vi "targeted_sensory_dynamics_v2.vi"() -> ()   [LabVIEW 2014]
uses:
  <vilib>/vision/Measure.llb/Straight Edge Options.ctl
  <vilib>/vision/Measure.llb/Straight Edge Process.ctl
  <vilib>/Platform/TimedLoop/XDataNode/timing_clust.ctl
  <vilib>/Platform/TimedLoop/XDataNode/nitl_modes.ctl
  <vilib>/Platform/TimedLoop/XDataNode/wakeup.ctl
  <vilib>/vision/Measure.llb/Edge Options.ctl
  <vilib>/vision/Measure.llb/Edge Polarity.ctl
  <vilib>/DAQmx/create/channels.llb/DAQmx Create Channel (DO-Digital Output).vi
  <vilib>/DAQmx/write.llb/DAQmx Write (Digital Bool 1Line 1Point).vi
  <vilib>/gmath/statdist.llb/Uniform (Discrete) Random.vi
  <vilib>/DAQmx/create/channels.llb/DAQmx Create Channel (AO-Voltage-Basic).vi
  <vilib>/Platform/TimedLoop/TimeConversion.llb/rt-rel-time-to-milliseconds.vi
  <vilib>/DAQmx/write.llb/DAQmx Write (Analog DBL 1Chan 1Samp).vi
  <vilib>/DAQmx/create/channels.llb/DAQmx Create Channel (DI-Digital Input).vi
  <vilib>/DAQmx/read.llb/DAQmx Read (Digital Bool 1Line 1Point).vi
  <vilib>/platform/TimedLoop/XDataNode/XDataNode.xnode
  <vilib>/vision/driver/NI_Vision_Acquisition_Software.lvlib
  <vilib>/Platform/TimedLoop/XDataNode/XDNodeRunTimeDep.lvlib
  <vilib>/vision/NI_Vision_Development_Module.lvlib
  <vilib>/gmath/NI_Gmath.lvlib
panel:
  out "Trial Light":dbl
  out "Light Trial?":bool=TRUE
  out "Slide 7":dbl(slide) scale=0.0..1.0
  out "Slide 6":dbl(slide) scale=0.0..1.0
  out "W, 90":i32
  out "M, 90":i32
  in  "Light Intensity (V)":dbl=3.9 format="%#_13g"
  in  "Wind Intensity (V)":dbl=3.7 format="%#_13g"
  out "Wind Trial?":bool=TRUE
  out "Initial Orientation":dbl
  out "Slide 5":dbl(slide) scale=0.0..1.0
  out "Slide 4":dbl(slide) scale=0.0..1.0
  out "Slide 3":dbl(slide) scale=0.0..1.0
  out "Slide 2":dbl(slide) scale=0.0..1.0
  out "V, 90":i32
  out "W, 0":i32
  out "M, 0":i32
  out "V, 0":i32
  in  "Reversed Tether?":bool=TRUE
  in  "R options":T1={"Number of Lines"=1, "Type"=enum."Best Edge Projection", "Min. Score"=10.0, "Max. Score"=1000.0, "Orientation"=-135.0, "Angle Range"=45.0, "Angle Tolerance"=1.0, "Step Size"=3, "Min. SNR (db)"=0.0, "Min. Points (%)"=25.0, "Hough Iterations"=3} {"Min. Points (%)" min=0.0 max=100.0; "Min. SNR (db)" min=0.0; "Max. Score" min=0.0 max=1024.0; "Min. Score" min=0.0 max=1024.0 step=1.0}
  in  "L options":T1={"Number of Lines"=1, "Type"=enum."Best Edge Projection", "Min. Score"=10.0, "Max. Score"=1000.0, "Orientation"=135.0, "Angle Range"=45.0, "Angle Tolerance"=1.0, "Step Size"=3, "Min. SNR (db)"=0.0, "Min. Points (%)"=25.0, "Hough Iterations"=3} {"Min. Points (%)" min=0.0 max=100.0; "Min. SNR (db)" min=0.0; "Max. Score" min=0.0 max=1024.0; "Min. Score" min=0.0 max=1024.0 step=1.0}
  out "X (steps/sample)":dbl(graph)
  out "Slide":dbl(slide) scale=0.0..1.0
  out "Motor Error":bool
  in  "Max steps/sample":dbl=6.0
  in  "Step Rate (Hz)":dbl=500.0
  out "Heading (deg)":dbl(graph)
  out "H":dbl format="%.4f"
  out "X (steps/sample)":dbl
  in  "Geneotype":string="w+ Canton-S"
  in  "Starvation Time (hrs)":string="1"
  in  "Age (DSE)":string="4"
  out "Trial End":bool
  in  "Trial Duration (s)":dbl=25.0
  out "Trial":i32 format="%#.3f"
  in  "Number of Trials":i32=30
  in  "Experiment name":string="E1"
  in  "Fly ID":string
  in  "L-R WBA Offset (deg)":dbl format="%#_13g"
  in  "deltaWBA Scale Factor (k, unitless)":dbl=0.04 format="%.4f"
  out "L-R WBA":dbl
  out "deltaWBA":dbl format="%.4f"
  out "Scaled deltaWBA (deg)":dbl(graph)
  out "R WBA":dbl
  out "L WBA":dbl
  out "Image":T3(plugin-control)
  in  "Image Threshold":cluster{"Lower value":sgl, "Upper value":sgl}={"Lower value"=110.0, "Upper value"=255.0} {"Upper value" format="%.2f"; "Lower value" format="%.2f"}
  in  "Data Rate (Hz)":dbl=50.0
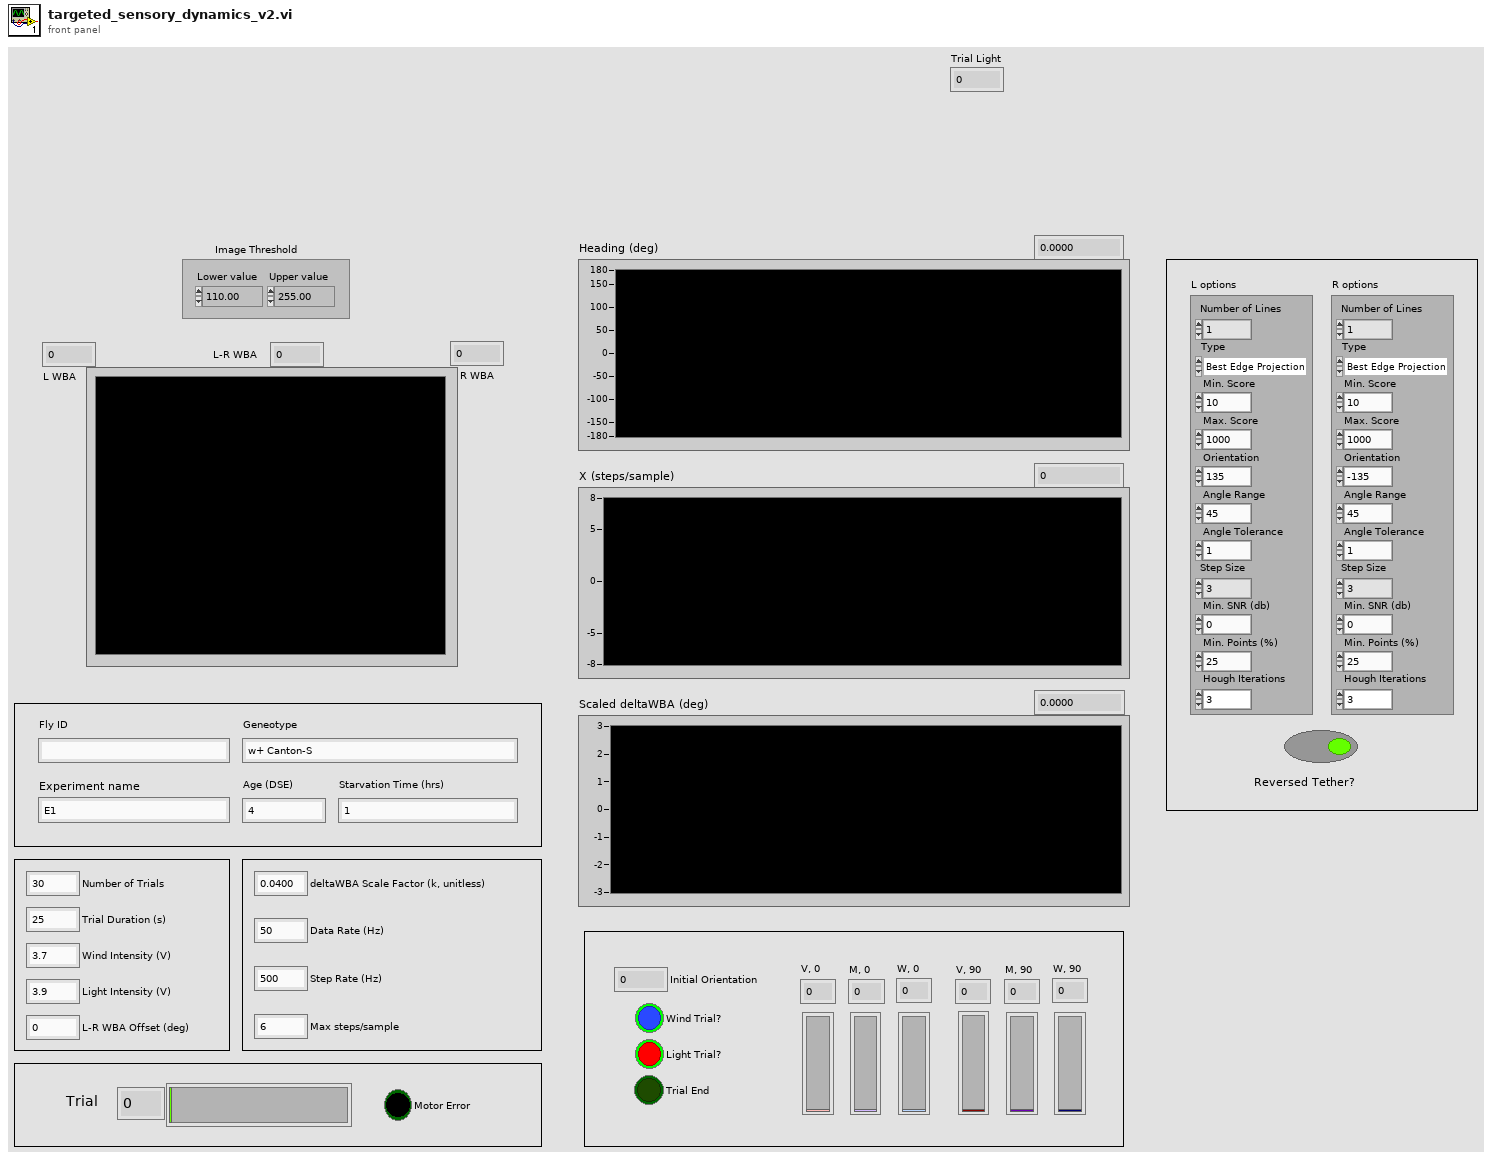
[diagram p1: front panel]
types:
  T1 = typedef "Straight Edge Options.ctl" = cluster{"Number of Lines":i32, "Type":T2, "Min. Score":dbl, "Max. Score":dbl, "Orientation":dbl, "Angle Range":dbl, "Angle Tolerance":dbl, "Step Size":u32, "Min. SNR (db)":dbl, "Min. Points (%)":dbl, "Hough Iterations":i32}
  T2 = typedef "Straight Edge Process.ctl" = enum32{"First Edge Rake", "Best Edge Rake", "Hough Edge Rake", "First Edge Projection", "Best Edge Projection"}
  T3 = typedef "IMAQ Image.ctl" = refnum<image>
  T4 = enum16{"open", "replace", "create", "open or create", "replace or create", "replace or create with confirmation"}
  T5 = typedef "IMAQdx.ctl" = refnum<k21>
  T6 = typedef "IMAQ Rectangle" = cluster{"Left":i32, "Top":i32, "Right":i32, "Bottom":i32, "Rotation":dbl}
  T7 = typedef "ROI Descriptor" = cluster{"Global Rectangle":i32[], "Contours":cluster{"ID":enum32{"External", "Internal"}, "Type":u32, "Coordinates":i32[]}[]}
  T8 = typedef "XDNodeRunTimeDep.lvlib/timing_clust.ctl" = cluster{"Expected End [f-1]":u64, "Actual End [f-1]":u64, "Finished Late? [f-1]":bool, "Expected End [i-1]":u64, "Actual End [i-1]":u64, "Finished Late? [i-1]":bool, "Expected Start [i]":u64, "Actual Start [i]":u64, "Expected Start [f]":u64, "Actual Start [f]":u64, "Source Name":string, "Structure Name":string, "Period":i64, "Deadline":i64, "Offset":i64, "Start":i64, "Priority":i32, "Timeout":i32, "Mode":T9, "Wakeup Reason":T10, "Error":errorcluster, "Source Type":string, "Secondary Source Type":string, "Global End Time":u64, "Global Start Time":u64, "Frame Duration":u64, "Iteration Duration":u64, "Assigned CPU":i32, "I/O Scan Engine Mode":u32}
  T9 = typedef "XDNodeRunTimeDep.lvlib/nitl_modes.ctl" = enum32{"No Change", "Process missed periods, maintain original phase", "Discard missed periods, maintain original phase", "Process missed periods, ignore original phase", "Discard missed periods, ignore original phase"}
  T10 = typedef "XDNodeRunTimeDep.lvlib/wakeup.ctl" = enum32{"Normal", "Aborted", "Asynchronous wakeup", "Timing source error", "Timed loop error", "Timeout"}
  T11 = cluster{"y":i32, "y":i32, "y":i32, "y":i32, "y":i32, "y":i32}
  T12 = typedef "Edge Options.ctl" = cluster{"Edge Polarity":T13, "Kernel Size":u32, "Width":u32, "Minimum Edge Strength":sgl, "Interpolation Type":enum32{"Zero Order", "Bilinear", "Quadratic", "Cubic", "Bilinear Fixed"}, "Data Processing Method":enum32{"Average", "Median"}}
  T13 = typedef "Edge Polarity.ctl" = u32
  T14 = cluster{"Search Direction":u32, "Edge Options":T12, "Show Search Area":bool, "Show Search Lines":bool, "Show Edges Found":bool, "Show Result":bool, "Search Area Color":u32, "Search Lines Color":u32, "Edge Locations Color":u32, "Result Color":u32, "Overlay Group Name":string}
  T15 = cluster{"Point1 (Pixels)":cluster{"X":sgl, "Y":sgl}, "Point2 (Pixels)":cluster{"X":sgl, "Y":sgl}, "Point1 (Real-World)":cluster{"X":sgl, "Y":sgl}, "Point2 (Real-World)":cluster{"X":sgl, "Y":sgl}, "Angle (Pixel)":dbl, "Angle (Real-World)":dbl, "Score":dbl, "Straightness":dbl, "Average SNR (db)":dbl, "Calibration Valid":bool}[]
  T16 = cluster{"Straight Edges[0]":cluster{"Point1 (Pixels)":cluster{"X":sgl, "Y":sgl}, "Point2 (Pixels)":cluster{"X":sgl, "Y":sgl}, "Point1 (Real-World)":cluster{"X":sgl, "Y":sgl}, "Point2 (Real-World)":cluster{"X":sgl, "Y":sgl}, "Angle (Pixel)":dbl, "Angle (Real-World)":dbl, "Score":dbl, "Straightness":dbl, "Average SNR (db)":dbl, "Calibration Valid":bool}, "Straight Edges[1]":cluster{"Point1 (Pixels)":cluster{"X":sgl, "Y":sgl}, "Point2 (Pixels)":cluster{"X":sgl, "Y":sgl}, "Point1 (Real-World)":cluster{"X":sgl, "Y":sgl}, "Point2 (Real-World)":cluster{"X":sgl, "Y":sgl}, "Angle (Pixel)":dbl, "Angle (Real-World)":dbl, "Score":dbl, "Straightness":dbl, "Average SNR (db)":dbl, "Calibration Valid":bool}, "Straight Edges[2]":cluster{"Point1 (Pixels)":cluster{"X":sgl, "Y":sgl}, "Point2 (Pixels)":cluster{"X":sgl, "Y":sgl}, "Point1 (Real-World)":cluster{"X":sgl, "Y":sgl}, "Point2 (Real-World)":cluster{"X":sgl, "Y":sgl}, "Angle (Pixel)":dbl, "Angle (Real-World)":dbl, "Score":dbl, "Straightness":dbl, "Average SNR (db)":dbl, "Calibration Valid":bool}, "Straight Edges[3]":cluster{"Point1 (Pixels)":cluster{"X":sgl, "Y":sgl}, "Point2 (Pixels)":cluster{"X":sgl, "Y":sgl}, "Point1 (Real-World)":cluster{"X":sgl, "Y":sgl}, "Point2 (Real-World)":cluster{"X":sgl, "Y":sgl}, "Angle (Pixel)":dbl, "Angle (Real-World)":dbl, "Score":dbl, "Straightness":dbl, "Average SNR (db)":dbl, "Calibration Valid":bool}, "Straight Edges[4]":cluster{"Point1 (Pixels)":cluster{"X":sgl, "Y":sgl}, "Point2 (Pixels)":cluster{"X":sgl, "Y":sgl}, "Point1 (Real-World)":cluster{"X":sgl, "Y":sgl}, "Point2 (Real-World)":cluster{"X":sgl, "Y":sgl}, "Angle (Pixel)":dbl, "Angle (Real-World)":dbl, "Score":dbl, "Straightness":dbl, "Average SNR (db)":dbl, "Calibration Valid":bool}, "Straight Edges[5]":cluster{"Point1 (Pixels)":cluster{"X":sgl, "Y":sgl}, "Point2 (Pixels)":cluster{"X":sgl, "Y":sgl}, "Point1 (Real-World)":cluster{"X":sgl, "Y":sgl}, "Point2 (Real-World)":cluster{"X":sgl, "Y":sgl}, "Angle (Pixel)":dbl, "Angle (Real-World)":dbl, "Score":dbl, "Straightness":dbl, "Average SNR (db)":dbl, "Calibration Valid":bool}, "Straight Edges[6]":cluster{"Point1 (Pixels)":cluster{"X":sgl, "Y":sgl}, "Point2 (Pixels)":cluster{"X":sgl, "Y":sgl}, "Point1 (Real-World)":cluster{"X":sgl, "Y":sgl}, "Point2 (Real-World)":cluster{"X":sgl, "Y":sgl}, "Angle (Pixel)":dbl, "Angle (Real-World)":dbl, "Score":dbl, "Straightness":dbl, "Average SNR (db)":dbl, "Calibration Valid":bool}, "Straight Edges[7]":cluster{"Point1 (Pixels)":cluster{"X":sgl, "Y":sgl}, "Point2 (Pixels)":cluster{"X":sgl, "Y":sgl}, "Point1 (Real-World)":cluster{"X":sgl, "Y":sgl}, "Point2 (Real-World)":cluster{"X":sgl, "Y":sgl}, "Angle (Pixel)":dbl, "Angle (Real-World)":dbl, "Score":dbl, "Straightness":dbl, "Average SNR (db)":dbl, "Calibration Valid":bool}, "Straight Edges[8]":cluster{"Point1 (Pixels)":cluster{"X":sgl, "Y":sgl}, "Point2 (Pixels)":cluster{"X":sgl, "Y":sgl}, "Point1 (Real-World)":cluster{"X":sgl, "Y":sgl}, "Point2 (Real-World)":cluster{"X":sgl, "Y":sgl}, "Angle (Pixel)":dbl, "Angle (Real-World)":dbl, "Score":dbl, "Straightness":dbl, "Average SNR (db)":dbl, "Calibration Valid":bool}}
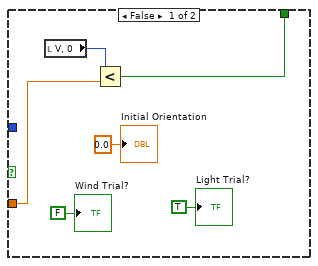
[diagram p2: hidden frame]
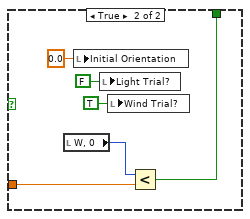
[diagram p3: hidden frame]
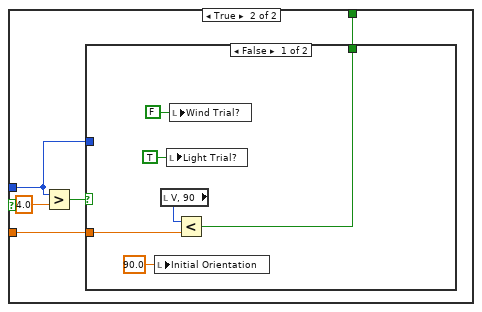
[diagram p4: hidden frame]
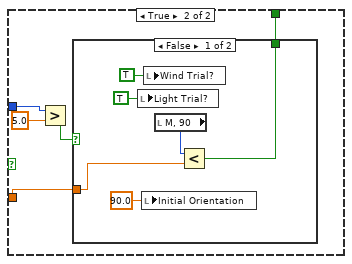
[diagram p5: hidden frame]
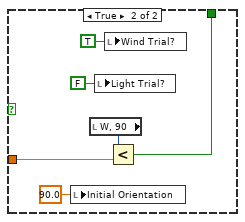
[diagram p6: hidden frame]
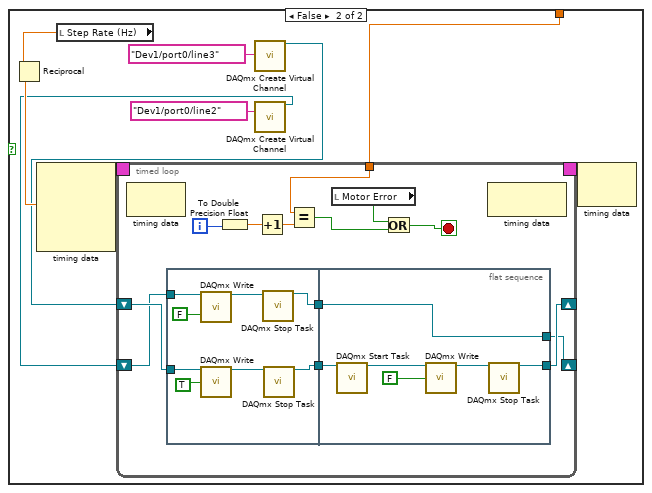
[diagram p8: hidden frame]
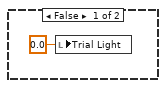
[diagram p9: hidden frame]
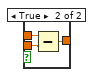
[diagram p11: hidden frame]
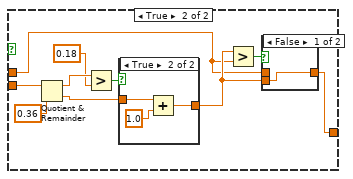
[diagram p15: hidden frame]
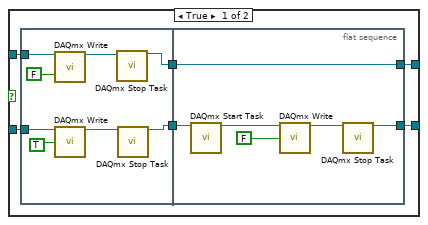
[diagram p19: hidden frame]
diagram:
  w83 = "."
  w85 = "."
  n1 = local read "Wind Intensity (V)"() -> (w21:dbl)
  n2 = local read "deltaWBA Scale Factor (k, unitless)"() -> (w63:dbl)
  n3 = local read "Data Rate (Hz)"() -> (w64:dbl)
  n4 = local read "Trial Duration (s)"() -> (w69:dbl)
  n5 = local read "Number of Trials"() -> (w71:i32)
  n6 = local read "Light Intensity (V)"() -> (w19:dbl)
  n7 = local read "Max steps/sample"() -> (w61:dbl)
  n8 = local read "Step Rate (Hz)"() -> (w62:dbl)
  n9 = local read "Reversed Tether?"() -> (w43:bool)
  n10 = Boolean To (0,1)(Boolean=w43) -> (0, 1=w44:i16)
  n11 = To Double Precision Float(number=w44) -> (double precision float=w42:dbl)
  n12 = Number To Fractional String(number=w19, precision (6)=i16 3) -> (F-format string=w17:string)  [unwired: 2 in]
  n13 = Number To Fractional String(number=w71, precision (6)=i16 0) -> (F-format string=w55:string)  [unwired: 2 in]
  n14 = Number To Fractional String(number=w69, precision (6)=i16 0) -> (F-format string=w54:string)  [unwired: 2 in]
  n15 = Number To Fractional String(number=w21, precision (6)=i16 3) -> (F-format string=w18:string)  [unwired: 2 in]
  n16 = Number To Fractional String(number=w64, precision (6)=i16 0) -> (F-format string=w16:string)  [unwired: 2 in]
  n17 = Number To Fractional String(number=w62, precision (6)=i16 0) -> (F-format string=w15:string)  [unwired: 2 in]
  n18 = Number To Fractional String(number=w61, precision (6)=i16 0) -> (F-format string=w14:string)  [unwired: 2 in]
  n19 = Number To Fractional String(number=w63, precision (6)=i16 3) -> (F-format string=w13:string)  [unwired: 2 in]
  n20 = Number To Fractional String(number=w42, precision (6)=i16 0) -> (F-format string=w12:string)  [unwired: 2 in]
  n21 = Get Date/Time In Seconds() -> (seconds since 1Jan1904=w91:timestamp)
  n22 = Get Date/Time In Seconds() -> (seconds since 1Jan1904=w87:timestamp)
  n23 = Get Date/Time In Seconds() -> (seconds since 1Jan1904=w89:timestamp)
  n24 = call <vilib>:"Space Constant.vi"() -> ("String"=w93:string)
  n25 = Format Date/Time String(time format string (%c)="%d", seconds (now)=w91) -> (date/time string=w82:string)  [unwired: 1 in]
  n26 = Format Date/Time String(time format string (%c)="%m", seconds (now)=w89) -> (date/time string=w84:string)  [unwired: 1 in]
  n27 = Format Date/Time String(time format string (%c)="%Y", seconds (now)=w87) -> (date/time string=w86:string)  [unwired: 1 in]
  n28 = Concatenate Strings(w86, w85, w84, w83, w82) -> (w60:string)
  n29 = Concatenate Strings(w86, w85, w84, w83, w82, w93, "fly_", "Fly ID", "\\") -> (w97:string)
  n30 = String To Path(string=w97) -> (path=w96:path)
  n31 = Build Path(base path=path "E:/TAC DATA ARCHIVE/NewRig/labview/ClosedLoop+OpenWindLightOdor", name or relative path=w96) -> (appended path=w101:path)
  n32 = call <vilib>:"IMAQdx Open Camera.vi"("Session In"=refnum<k21> "cam8" ("Camera Name")) -> ("Session Out"=w123:T5)  [unwired: 2 in, 8 out]
  n33 = call <vilib>:"Check if File or Folder Exists.vi"("path"=w101) -> ("file or folder exists?"=w99:bool, "dup path"=w100:path)  [unwired: 8 in, 1 out]
  n34 = call <vilib>:"IMAQdx Configure Grab.vi"("Session In"=w123) -> ("Session Out"=w121:T5)  [unwired: 1 in, 9 out]
  n35 = case shown="False" w99 {
    tunnel: w100 -> [w125 w126]
    tunnel: [w124 w126] -> w105
    frame False {
      n36 = Create Folder(path (use dialog)=w125) -> (created path=w124:path)  [unwired: 2 in, 2 out]
    }
    frame True {
    }
  }
  n37 = call "IMAQ Create"("Image Name"="ROIR") -> ("New Image"=w120:T3)  [unwired: 3 in, 2 out]
  n38 = Concatenate Strings("Experiment name", "\\") -> (w73:string)
  n39 = call <vilib>:"IMAQdx Grab.vi"("Image In"=w120, "Session In"=w121) -> ("Image Out"=w119:T3, "Session Out"=w110:T5)  [unwired: 2 in, 6 out]
  n40 = String To Path(string=w73) -> (path=w102:path)
  n41 = call "IMAQ Select Rectangle"("Prompt"="Select RIGHT ROI for wing angle detection", "Image In"=w119) -> ("Rectangle"=w111:T6)  [unwired: 6 in, 3 out]
  n42 = Build Path(base path=w105, name or relative path=w102) -> (appended path=w106:path)
  n43 = call "IMAQ Convert Rectangle to ROI"("Rectangle"=w111) -> ("ROI Descriptor"=w109:T7)  [unwired: 8 in, 1 out]
  n44 = call <vilib>:"Check if File or Folder Exists.vi"("path"=w106) -> ("file or folder exists?"=w103:bool, "dup path"=w104:path)  [unwired: 8 in, 1 out]
  n45 = call "IMAQ Create"("Image Name"="ROIL") -> ("New Image"=w115:T3)  [unwired: 3 in, 2 out]
  n46 = case shown="False" w103 {
    tunnel: w104 -> [w128 w129]
    tunnel: [w127 w129] -> w6
    frame False {
      n47 = Create Folder(path (use dialog)=w128) -> (created path=w127:path)  [unwired: 2 in, 2 out]
    }
    frame True {
    }
  }
  n48 = call <vilib>:"IMAQdx Grab.vi"("Image In"=w115, "Session In"=w110) -> ("Image Out"=w114:T3, "Session Out"=w108:T5)  [unwired: 2 in, 6 out]
  n49 = String To Path(string="experiment_information") -> (path=w81:path)
  n50 = call "IMAQ Select Rectangle"("Prompt"="Select LEFT ROI for wing angle detection", "Image In"=w114) -> ("Rectangle"=w116:T6)  [unwired: 6 in, 3 out]
  n51 = Build Path(base path=w6, name or relative path=w81) -> (appended path=w78:path)
  n52 = String To Path(string="initial_orientations") -> (path=w31:path)
  n53 = String To Path(string="wind_boolean") -> (path=w52:path)
  n54 = String To Path(string="light_boolean") -> (path=w10:path)
  n55 = call "IMAQ Convert Rectangle to ROI"("Rectangle"=w116) -> ("ROI Descriptor"=w107:T7)  [unwired: 8 in, 1 out]
  n56 = Build Path(base path=w6, name or relative path=w31) -> (appended path=w28:path)
  n57 = Build Path(base path=w6, name or relative path=w52) -> (appended path=w49:path)
  n58 = Build Path(base path=w6, name or relative path=w10) -> (appended path=w8:path)
  n59 = Open/Create/Replace File(file path (use dialog)=w78, operation (0:open)=T4."create", access (0:read/write)=enum16{"read/write", "read-only", "write-only"}."write-only") -> (refnum out=w76:refnum<file>)  [unwired: 3 in, 2 out]
  n60 = Open/Create/Replace File(file path (use dialog)=w28, operation (0:open)=T4."create", access (0:read/write)=enum16{"read/write", "read-only", "write-only"}."write-only") -> (refnum out=w26:refnum<file>)  [unwired: 3 in, 2 out]
  n61 = Open/Create/Replace File(file path (use dialog)=w49, operation (0:open)=T4."create", access (0:read/write)=enum16{"read/write", "read-only", "write-only"}."write-only") -> (refnum out=w47:refnum<file>)  [unwired: 3 in, 2 out]
  n62 = Open/Create/Replace File(file path (use dialog)=w8, operation (0:open)=T4."create", access (0:read/write)=enum16{"read/write", "read-only", "write-only"}."write-only") -> (refnum out=w5:refnum<file>)  [unwired: 3 in, 2 out]
  n63 = Build Array(w60, "Fly ID", "Experiment name", "Age (DSE)", "Starvation Time (hrs)", w55, w54, w18, w17, w16, w15, w14, w13, w12, "Geneotype") -> (w53:string[])
  n64 = Write to Text File(file (use dialog)=w76, text=w53) -> (refnum out=w75:refnum<file>)  [unwired: 2 in, 2 out]
  n65 = Close File(refnum=w75) -> ()  [unwired: 1 in, 2 out]
  n66 = flat-sequence {
    tunnel: w6 -> [w134]
    tunnel: w107 -> [w135]
    tunnel: w108 -> [w136]
    tunnel: w109 -> [w137]
    tunnel: [w137] -> w41
    tunnel: [w136] -> w39
    tunnel: [w135] -> w37
    tunnel: [w134] -> w35
    tunnel: [w132] -> w33
    tunnel: w47 -> [w132]
    tunnel: w26 -> [w131]
    tunnel: [w131] -> w24
    tunnel: w5 -> [w130]
    tunnel: [w130] -> w3
    tunnel: w41 -> [w144]
    tunnel: [w144] -> w40
    tunnel: w39 -> [w143]
    tunnel: [w143] -> w38
    tunnel: w37 -> [w142]
    tunnel: [w142] -> w36
    tunnel: w35 -> [w141]
    tunnel: [w141] -> w34
    tunnel: w33 -> [w140]
    tunnel: [w140] -> w32
    tunnel: [w139] -> w25
    tunnel: w24 -> [w139]
    tunnel: [w138] -> w4
    tunnel: w3 -> [w138]
    tunnel: w40 -> [w161]
    tunnel: w38 -> [w160]
    tunnel: w36 -> [w159]
    tunnel: w34 -> [w158]
    tunnel: w32 -> [w156]
    tunnel: [w155] -> w46
    tunnel: w25 -> [w150]
    tunnel: [w149] -> w23
    tunnel: w4 -> [w146]
    tunnel: [w145] -> w2
    tunnel: w46 -> [w1061]
    tunnel: w23 -> [w1055]
    tunnel: w2 -> [w1054]
    frame #0 {
      n67 = One Button Dialog(message="Ensure the stage is at 0 degrees.") -> ()  [unwired: 1 in, 1 out]
    }
    frame #1 {
    }
    frame #2 {
      n68 = for {
        N: "Number of Trials" -> [_]
        tunnel: w161 -> [w250]
        tunnel: w160 -> [w249]
        tunnel: w159 -> [w248]
        tunnel: w158 -> [w247]
        shift-right: [w226] -> w155
        shift-left: w156 -> [w230]
        shift-right: [w221] -> _
        shift-left: 0 ("y") -> [w215]
        shift-right: [w220] -> _
        shift-left: 0 ("y") -> [w213]
        shift-right: [w219] -> _
        shift-left: 0 ("y") -> [w211]
        shift-right: [w218] -> _
        shift-left: 0 ("y") -> [w209]
        shift-right: [w178] -> w149
        shift-left: w150 -> [w184]
        shift-right: [w169] -> _
        shift-left: 0 ("y") -> [w173]
        shift-right: [w170] -> _
        shift-left: 0 ("y") -> [w174]
        shift-right: [w162] -> w145
        shift-left: w146 -> [w168]
        i -> [w244]
        n69 = local read "Number of Trials"() -> (w217:i32)
        n70 = local read "Number of Trials"() -> (w235:i32)
        n71 = Divide(x=w217, y=6) -> (x/y=w175:dbl)
        n72 = Divide(x=w215, y=w175) -> (x/y=→"Slide 2":dbl)
        n73 = Divide(x=w173, y=w175) -> (x/y=→"Slide 6":dbl)
        n74 = Divide(x=w211, y=w175) -> (x/y=→"Slide 4":dbl)
        n75 = Divide(x=w213, y=w175) -> (x/y=→"Slide 3":dbl)
        n76 = Divide(x=w209, y=w175) -> (x/y=→"Slide 5":dbl)
        n77 = Divide(x=w174, y=w175) -> (x/y=→"Slide 7":dbl)
        n78 = flat-sequence {
          tunnel: w234 -> [w274]
          tunnel: w247 -> [w275]
          tunnel: w248 -> [w276]
          tunnel: w249 -> [w277]
          tunnel: w250 -> [w278]
          tunnel: [w278] -> w207
          tunnel: [w277] -> w205
          tunnel: [w276] -> w203
          tunnel: [w275] -> w201
          tunnel: [w274] -> w199
          tunnel: w230 -> [w266]
          tunnel: [w266] -> w197
          tunnel: [w265] -> w195
          tunnel: w211 -> [w262]
          tunnel: w209 -> [w261]
          tunnel: w213 -> [w263]
          tunnel: w215 -> [w264]
          tunnel: w175 -> [w260]
          tunnel: [w264] -> w193
          tunnel: [w263] -> w192
          tunnel: [w262] -> w191
          tunnel: [w261] -> w190
          tunnel: w184 -> [w259]
          tunnel: [w259] -> w183
          tunnel: w173 -> [w258]
          tunnel: w174 -> [w257]
          tunnel: [w258] -> w172
          tunnel: [w257] -> w171
          tunnel: w168 -> [w256]
          tunnel: [w256] -> w166
          tunnel: w207 -> [w363]
          tunnel: [w363] -> w206
          tunnel: w205 -> [w362]
          tunnel: [w362] -> w204
          tunnel: w203 -> [w361]
          tunnel: [w361] -> w202
          tunnel: w201 -> [w360]
          tunnel: [w360] -> w200
          tunnel: w199 -> [w359]
          tunnel: [w359] -> w198
          tunnel: w197 -> [w358]
          tunnel: [w358] -> w196
          tunnel: w195 -> [w350]
          tunnel: [w357] -> w194
          tunnel: w193 -> [w356]
          tunnel: w192 -> [w355]
          tunnel: w191 -> [w354]
          tunnel: w190 -> [w353]
          tunnel: [w351] -> w189
          tunnel: [w350] -> w188
          tunnel: w183 -> [w349]
          tunnel: [w348] -> w182
          tunnel: w172 -> [w346]
          tunnel: w171 -> [w345]
          tunnel: [w344] -> w167
          tunnel: w166 -> [w344]
          tunnel: [w449] -> w255
          tunnel: [w448] -> w254
          tunnel: [w447] -> w253
          tunnel: [w416] -> w252
          tunnel: w206 -> [w449]
          tunnel: w204 -> [w448]
          tunnel: w202 -> [w447]
          tunnel: w200 -> [w393]
          tunnel: w198 -> [w392]
          tunnel: [w415] -> w243
          tunnel: [w414] -> w240
          tunnel: [w391] -> w239
          tunnel: [w390] -> w238
          tunnel: [w389] -> w232
          tunnel: w196 -> [w388]
          tunnel: [w386] -> w229
          tunnel: w194 -> [w385]
          tunnel: [w385] -> w224
          tunnel: w189 -> [w384]
          tunnel: w188 -> [w371]
          tunnel: [w371] -> w187
          tunnel: w182 -> [w370]
          tunnel: [w370] -> w181
          tunnel: w167 -> [w365]
          tunnel: [w364] -> w165
          tunnel: w255 -> [w584]
          tunnel: w254 -> [w583]
          tunnel: w253 -> [w582]
          tunnel: w252 -> [w581]
          tunnel: [w580] -> w251
          tunnel: [w579] -> w246
          tunnel: [w578] -> w245
          tunnel: w243 -> [w577]
          tunnel: [w576] -> w242
          tunnel: [w575] -> w241
          tunnel: w240 -> [w574]
          tunnel: w239 -> [w573]
          tunnel: w238 -> [w572]
          tunnel: [w571] -> w237
          tunnel: [w570] -> w236
          tunnel: w232 -> [w563]
          tunnel: [w560] -> w231
          tunnel: w229 -> [w559]
          tunnel: [w559] -> w228
          tunnel: [w556] -> w225
          tunnel: w224 -> [w555]
          tunnel: [w555] -> w223
          tunnel: w187 -> [w554]
          tunnel: [w554] -> w186
          tunnel: w181 -> [w553]
          tunnel: [w553] -> w179
          tunnel: w165 -> [w552]
          tunnel: [w552] -> w164
          tunnel: w251 -> [w818]
          tunnel: w246 -> [w821]
          tunnel: w245 -> [w820]
          tunnel: w242 -> [w819]
          tunnel: w241 -> [w817]
          tunnel: w237 -> [w816]
          tunnel: w236 -> [w815]
          tunnel: w231 -> [w811]
          tunnel: w228 -> [w808]
          tunnel: [w808] -> w227
          tunnel: w225 -> [w804]
          tunnel: w223 -> [w802]
          tunnel: [w802] -> w222
          tunnel: w186 -> [w799]
          tunnel: [w799] -> w185
          tunnel: [w798] -> w180
          tunnel: w179 -> [w798]
          tunnel: w164 -> [w797]
          tunnel: [w797] -> w163
          tunnel: w227 -> [w946]
          tunnel: [w946] -> w226
          tunnel: w222 -> [w945]
          tunnel: [w944] -> w221
          tunnel: [w943] -> w220
          tunnel: [w942] -> w219
          tunnel: [w941] -> w218
          tunnel: w185 -> [w935]
          tunnel: [w934] -> w178
          tunnel: w180 -> [w934]
          tunnel: [w930] -> w169
          tunnel: [w929] -> w170
          tunnel: w163 -> [w928]
          tunnel: [w928] -> w162
          frame #0 {
            n79 = while {
              tunnel: w260 -> [w280]
              tunnel: [w281] -> w265
              stop <- w279 stop-if-true
              n80 = call-poly <vilib>:"Discrete Random.vi"("n"=6, "samples"=1) -> ("uniform (discrete) random data"=w284:i32[])  [unwired: 8 in, 1 out]
              n81 = Index Array(array=w284, index=0) -> (element=w281:i32)
              n82 = Greater?(x=w281, y=3.0) -> (0:w282:bool)
              n83 = case shown="False" w282 {
                tunnel: w281 -> [w288 w316]
                tunnel: w280 -> [w290 w318]
                tunnel: [w289 w317] -> w279
                frame False {
                  n84 = Greater?(x=w288, y=1.0) -> (0:w291:bool)
                  n85 = case shown="True" w291 {
                    tunnel: w290 -> [w297 w303]
                    tunnel: [w296 w302] -> w289
                    tunnel: w288 -> [_ w299]
                    frame False {
                      n86 = local read "V, 0"() -> (w298:i32)
                      n87 = Less?(x=w298, y=w297) -> (x < y?=w296:bool)
                      "Initial Orientation" <- 0.0
                      "Wind Trial?" <- FALSE ("Win Trial?")
                      "Light Trial?" <- TRUE ("Light Trial?")
                    }
                    frame True {
                      n88 = Greater?(x=w299, y=2.0) -> (0:w300:bool)
                      n89 = case shown="False" w300 {
                        tunnel: w303 -> [w308 w314]
                        tunnel: [w307 w313] -> w302
                        frame False {
                          n90 = local write "Initial Orientation"(0.0 ("Initial Orientation")) -> ()
                          n91 = local write "Wind Trial?"(TRUE ("Wind Trial?")) -> ()
                          n92 = local write "Light Trial?"(TRUE ("Light Trial?")) -> ()
                          n93 = local read "M, 0"() -> (w309:i32)
                          n94 = Less?(x=w309, y=w308) -> (x < y?=w307:bool)
                        }
                        frame True {
                          n95 = local read "W, 0"() -> (w315:i32)
                          n96 = local write "Initial Orientation"(0.0 ("Initial Orientation")) -> ()
                          n97 = local write "Light Trial?"(FALSE ("Light Trial?")) -> ()
                          n98 = local write "Wind Trial?"(TRUE ("Wind Trial?")) -> ()
                          n99 = Less?(x=w315, y=w314) -> (x < y?=w313:bool)
                        }
                      }
                    }
                  }
                }
                frame True {
                  n100 = Greater?(x=w316, y=4.0) -> (0:w319:bool)
                  n101 = case shown="False" w319 {
                    tunnel: w318 -> [w325 w331]
                    tunnel: [w324 w330] -> w317
                    tunnel: w316 -> [_ w327]
                    frame False {
                      n102 = local write "Initial Orientation"(90.0 ("Light Intensity (V)")) -> ()
                      n103 = local read "V, 90"() -> (w326:i32)
                      n104 = local write "Light Trial?"(TRUE ("Light Trial?")) -> ()
                      n105 = local write "Wind Trial?"(FALSE ("Wind Trial?")) -> ()
                      n106 = Less?(x=w326, y=w325) -> (x < y?=w324:bool)
                    }
                    frame True {
                      n107 = Greater?(x=w327, y=5.0) -> (0:w328:bool)
                      n108 = case shown="False" w328 {
                        tunnel: w331 -> [w336 w342]
                        tunnel: [w335 w341] -> w330
                        frame False {
                          n109 = local write "Light Trial?"(TRUE ("Light Trial?")) -> ()
                          n110 = local write "Initial Orientation"(90.0 ("Initial Orientation")) -> ()
                          n111 = local write "Wind Trial?"(TRUE ("Wind Trial?")) -> ()
                          n112 = local read "M, 90"() -> (w337:i32)
                          n113 = Less?(x=w337, y=w336) -> (x < y?=w335:bool)
                        }
                        frame True {
                          n114 = local write "Initial Orientation"(90.0 ("Light Intensity (V)")) -> ()
                          n115 = local read "W, 90"() -> (w343:i32)
                          n116 = local write "Light Trial?"(FALSE ("Light Trial?")) -> ()
                          n117 = local write "Wind Trial?"(TRUE ("Wind Trial?")) -> ()
                          n118 = Less?(x=w343, y=w342) -> (x < y?=w341:bool)
                        }
                      }
                    }
                  }
                }
              }
            }
            n119 = local write "Motor Error"(FALSE ("Trial End")) -> ()
            n120 = call-poly <vilib>:"DAQmx Create Virtual Channel.vi"("lines"=tag "Dev1/port0/line0") -> ("task out"=w272:refnum<k21>)  [unwired: 13 in, 1 out]
            n121 = local write "Trial End"(FALSE ("Trial End")) -> ()
            n122 = call <vilib>:"DAQmx Start Task.vi"("task/channels in"=w272) -> ("task out"=w271:refnum<k21>)  [unwired: 13 in, 1 out]
            n123 = call-poly <vilib>:"DAQmx Write.vi"("task/channels in"=w271, "data"=FALSE) -> ("task out"=w270:refnum<k21>)  [unwired: 11 in, 2 out]
            n124 = call <vilib>:"DAQmx Stop Task.vi"("task/channels in"=w270) -> ()  [unwired: 13 in, 2 out]
          }
          frame #1 {
            n125 = local read "Initial Orientation"() -> (w347:dbl)
            n126 = Write to Binary File(file (use dialog)=w349, data=w347) -> (refnum out=w348:refnum<file>)  [unwired: 4 in, 2 out]
            n127 = call-poly <vilib>:"DAQmx Create Virtual Channel.vi"("physical channels"=tag "Dev1/ao1") -> ("task out"=w351:refnum<k21>)  [unwired: 13 in, 1 out]
            n128 = Bundle("y"=w356, "y"=w355, "y"=w354, "y"=w353, "y"=w346, "y"=w345) -> (w357:T11)  [unwired: 1 in]
          }
          frame #2 {
            n129 = local read "Initial Orientation"() -> (w373:dbl)
            n130 = flat-sequence {
              tunnel: ["Wind Intensity (V)"] -> w383
              tunnel: [w539] -> w369
              tunnel: ["Light Intensity (V)"] -> w368
              tunnel: w384 -> [w545]
              tunnel: w383 -> [w543]
              tunnel: w369 -> [w542]
              tunnel: w368 -> [w541]
              frame #0 {
                n131 = local read "Light Trial?"() -> (w539:bool)
              }
              frame #1 {
                n132 = Greater Than 0?(x=w543) -> (x > 0?=w544:bool)
                n133 = case shown="True" w542 {
                  tunnel: w541 -> [_ w547]
                  frame False {
                    n134 = local write "Trial Light"(0.0 ("Trial Light")) -> ()
                  }
                  frame True {
                    "Trial Light" <- w547
                  }
                }
                n135 = case shown="True" w544 {
                  tunnel: w545 -> [_ w551]
                  tunnel: w543 -> [_ w548]
                  frame False {
                  }
                  frame True {
                    n136 = call <vilib>:"DAQmx Start Task.vi"("task/channels in"=w551) -> ("task out"=w550:refnum<k21>)  [unwired: 13 in, 1 out]
                    n137 = call-poly <vilib>:"DAQmx Write.vi"("task/channels in"=w550, "data"=w548) -> ("task out"=w549:refnum<k21>)  [unwired: 11 in, 2 out]
                    n138 = call <vilib>:"DAQmx Stop Task.vi"("task/channels in"=w549) -> ()  [unwired: 13 in, 2 out]
                  }
                }
              }
            }
            n139 = call <vilib>:"Space Constant.vi"() -> ("String"=w419:string)
            n140 = call <vilib>:"Space Constant.vi"() -> ("String"=w439:string)
            n141 = call <vilib>:"Space Constant.vi"() -> ("String"=w406:string)
            n142 = call <vilib>:"Space Constant.vi"() -> ("String"=w430:string)
            n143 = call <vilib>:"Space Constant.vi"() -> ("String"=w396:string)
            n144 = Number To Fractional String(number=w392, precision (6)=i16 0) -> (F-format string=w422:string)  [unwired: 2 in]
            n145 = Number To Fractional String(number=w392, precision (6)=i16 0) -> (F-format string=w442:string)  [unwired: 2 in]
            n146 = Number To Fractional String(number=w392, precision (6)=i16 0) -> (F-format string=w409:string)  [unwired: 2 in]
            n147 = Number To Fractional String(number=w392, precision (6)=i16 0) -> (F-format string=w433:string)  [unwired: 2 in]
            n148 = Number To Fractional String(number=w392, precision (6)=i16 0) -> (F-format string=w399:string)  [unwired: 2 in]
            n149 = Concatenate Strings("trial", w419, w422, w419, "x_data") -> (w424:string)
            n150 = Concatenate Strings("trial", w439, w442, w439, "heading_data") -> (w444:string)
            n151 = Concatenate Strings("trial", w406, w409, w406, "LWBA_data") -> (w411:string)
            n152 = Concatenate Strings("trial", w430, w433, w430, "unfiltered deltaWBA") -> (w435:string)
            n153 = Concatenate Strings("trial", w396, w399, w396, "RWBA_data") -> (w401:string)
            n154 = local read "Wind Trial?"() -> (w372:bool)
            n155 = String To Path(string=w424) -> (path=w425:path)
            n156 = Divide(x=w373, y=0.36) -> (x/y=w381:dbl)
            n157 = String To Path(string=w444) -> (path=w445:path)
            n158 = String To Path(string=w411) -> (path=w412:path)
            n159 = String To Path(string=w435) -> (path=w436:path)
            n160 = String To Path(string=w401) -> (path=w402:path)
            n161 = local read "Light Trial?"() -> (w366:bool)
            n162 = To Long Integer(number=w381) -> (32bit integer=w374:i32)
            n163 = Greater Than 0?(x=w374) -> (x > 0?=w380:bool)
            n164 = Not Equal To 0?(x=w374) -> (x != 0?=w375:bool)
            n165 = Build Path(base path=w393, name or relative path=w425) -> (appended path=w418:path)
            n166 = Build Path(base path=w393, name or relative path=w445) -> (appended path=w438:path)
            n167 = Build Path(base path=w393, name or relative path=w412) -> (appended path=w405:path)
            n168 = Build Path(base path=w393, name or relative path=w436) -> (appended path=w429:path)
            n169 = Build Path(base path=w393, name or relative path=w402) -> (appended path=w395:path)
            n170 = To Double Precision Float(number=w374) -> (double precision float=w377:dbl)
            n171 = Absolute Value(x=w374) -> (abs(x)=w379:i32)
            n172 = Boolean To (0,1)(Boolean=w372) -> (0, 1=w387:i16)
            n173 = Multiply(x=0.36, y=w377) -> (x*y=w389:dbl)
            n174 = To Double Precision Float(number=w379) -> (double precision float=w378:dbl)
            n175 = case shown="True" w375 {
              tunnel: w380 -> [_ w451]
              tunnel: w378 -> [_ w450]
              frame False {
              }
              frame True {
                n176 = case shown="True" w451 {
                  tunnel: w450 -> [w452 w495]
                  frame True {
                    n177 = local read "Step Rate (Hz)"() -> (w455:dbl)
                    n178 = Reciprocal(x=w455) -> (1/x=w456:dbl)
                    n179 = node-c288(w456) -> (w458:T8)  [unwired: 3 in]
                    n180 = call-poly <vilib>:"DAQmx Create Virtual Channel.vi"("lines"=tag "Dev1/port0/line3") -> ("task out"=w454:refnum<k21>)  [unwired: 13 in, 1 out]
                    n181 = call-poly <vilib>:"DAQmx Create Virtual Channel.vi"("lines"=tag "Dev1/port0/line2") -> ("task out"=w453:refnum<k21>)  [unwired: 13 in, 1 out]
                    n182 = timed-loop {
                      timing: w458 -> [_]
                      timing-out: [_] -> w457
                      shift-right: [w471] -> _
                      shift-left: w454 -> [w469]
                      shift-right: [w470] -> _
                      shift-left: w453 -> [w468]
                      tunnel: w452 -> [w465]
                      i -> [w464]
                      stop <- w463 stop-if-true
                      n183 = node-c288() -> ()  [unwired: 1 in, 1 out]
                      n184 = flat-sequence {
                        tunnel: [w478] -> w473
                        tunnel: [w476] -> w472
                        tunnel: w469 -> [w475]
                        tunnel: w468 -> [w474]
                        tunnel: [w487] -> w471
                        tunnel: [w483] -> w470
                        tunnel: w473 -> [w486]
                        tunnel: w472 -> [w487]
                        frame #0 {
                          n185 = call-poly <vilib>:"DAQmx Write.vi"("task/channels in"=w475, "data"=FALSE) -> ("task out"=w477:refnum<k21>)  [unwired: 11 in, 2 out]
                          n186 = call-poly <vilib>:"DAQmx Write.vi"("task/channels in"=w474, "data"=TRUE) -> ("task out"=w479:refnum<k21>)  [unwired: 11 in, 2 out]
                          n187 = call <vilib>:"DAQmx Stop Task.vi"("task/channels in"=w477) -> ("task out"=w476:refnum<k21>)  [unwired: 13 in, 1 out]
                          n188 = call <vilib>:"DAQmx Stop Task.vi"("task/channels in"=w479) -> ("task out"=w478:refnum<k21>)  [unwired: 13 in, 1 out]
                        }
                        frame #1 {
                          n189 = call <vilib>:"DAQmx Start Task.vi"("task/channels in"=w486) -> ("task out"=w485:refnum<k21>)  [unwired: 13 in, 1 out]
                          n190 = call-poly <vilib>:"DAQmx Write.vi"("task/channels in"=w485, "data"=FALSE) -> ("task out"=w484:refnum<k21>)  [unwired: 11 in, 2 out]
                          n191 = call <vilib>:"DAQmx Stop Task.vi"("task/channels in"=w484) -> ("task out"=w483:refnum<k21>)  [unwired: 13 in, 1 out]
                        }
                      }
                      n192 = To Double Precision Float(number=w464) -> (double precision float=w466:dbl)
                      n193 = Increment(x=w466) -> (x+1=w467:dbl)
                      n194 = local read "Motor Error"() -> (w461:bool)
                      n195 = Equal?(x=w465, y=w467) -> (x = y?=w462:bool)
                      n196 = Or(x=w461, y=w462) -> (x .or. y?=w463:bool)
                      n197 = node-c288() -> ()  [unwired: 1 in, 1 out]
                    }
                    n198 = node-c288(w457) -> ()  [unwired: 1 out]
                  }
                  frame False {
                    n199 = local read "Step Rate (Hz)"() -> (w498:dbl)
                    n200 = Reciprocal(x=w498) -> (1/x=w499:dbl)
                    n201 = node-c288(w499) -> (w501:T8)  [unwired: 3 in]
                    n202 = call-poly <vilib>:"DAQmx Create Virtual Channel.vi"("lines"=tag "Dev1/port0/line3") -> ("task out"=w497:refnum<k21>)  [unwired: 13 in, 1 out]
                    n203 = call-poly <vilib>:"DAQmx Create Virtual Channel.vi"("lines"=tag "Dev1/port0/line2") -> ("task out"=w496:refnum<k21>)  [unwired: 13 in, 1 out]
                    n204 = timed-loop {
                      timing: w501 -> [_]
                      timing-out: [_] -> w500
                      shift-right: [w513] -> _
                      shift-left: w497 -> [w514]
                      shift-right: [w511] -> _
                      shift-left: w496 -> [w512]
                      tunnel: w495 -> [w507]
                      i -> [w506]
                      stop <- w505 stop-if-true
                      n205 = node-c288() -> ()  [unwired: 1 in, 1 out]
                      n206 = flat-sequence {
                        tunnel: [w521] -> w516
                        tunnel: [w519] -> w515
                        tunnel: w512 -> [w518]
                        tunnel: w514 -> [w517]
                        tunnel: [w530] -> w511
                        tunnel: [w526] -> w513
                        tunnel: w516 -> [w529]
                        tunnel: w515 -> [w530]
                        frame #0 {
                          n207 = call-poly <vilib>:"DAQmx Write.vi"("task/channels in"=w518, "data"=FALSE) -> ("task out"=w520:refnum<k21>)  [unwired: 11 in, 2 out]
                          n208 = call-poly <vilib>:"DAQmx Write.vi"("task/channels in"=w517, "data"=TRUE) -> ("task out"=w522:refnum<k21>)  [unwired: 11 in, 2 out]
                          n209 = call <vilib>:"DAQmx Stop Task.vi"("task/channels in"=w520) -> ("task out"=w519:refnum<k21>)  [unwired: 13 in, 1 out]
                          n210 = call <vilib>:"DAQmx Stop Task.vi"("task/channels in"=w522) -> ("task out"=w521:refnum<k21>)  [unwired: 13 in, 1 out]
                        }
                        frame #1 {
                          n211 = call <vilib>:"DAQmx Start Task.vi"("task/channels in"=w529) -> ("task out"=w528:refnum<k21>)  [unwired: 13 in, 1 out]
                          n212 = call-poly <vilib>:"DAQmx Write.vi"("task/channels in"=w528, "data"=FALSE) -> ("task out"=w527:refnum<k21>)  [unwired: 11 in, 2 out]
                          n213 = call <vilib>:"DAQmx Stop Task.vi"("task/channels in"=w527) -> ("task out"=w526:refnum<k21>)  [unwired: 13 in, 1 out]
                        }
                      }
                      n214 = To Double Precision Float(number=w506) -> (double precision float=w509:dbl)
                      n215 = Increment(x=w509) -> (x+1=w510:dbl)
                      n216 = Equal?(x=w507, y=w510) -> (x = y?=w508:bool)
                      n217 = local read "Motor Error"() -> (w504:bool)
                      n218 = Or(x=w504, y=w508) -> (x .or. y?=w505:bool)
                      n219 = node-c288() -> ()  [unwired: 1 in, 1 out]
                    }
                    n220 = node-c288(w500) -> ()  [unwired: 1 out]
                  }
                }
              }
            }
            n221 = Boolean To (0,1)(Boolean=w366) -> (0, 1=w367:i16)
            n222 = Open/Create/Replace File(file path (use dialog)=w418, operation (0:open)=T4."create", access (0:read/write)=enum16{"read/write", "read-only", "write-only"}."write-only") -> (refnum out=w416:refnum<file>)  [unwired: 3 in, 2 out]
            n223 = Open/Create/Replace File(file path (use dialog)=w438, operation (0:open)=T4."create", access (0:read/write)=enum16{"read/write", "read-only", "write-only"}."write-only") -> (refnum out=w415:refnum<file>)  [unwired: 3 in, 2 out]
            n224 = Open/Create/Replace File(file path (use dialog)=w405, operation (0:open)=T4."create", access (0:read/write)=enum16{"read/write", "read-only", "write-only"}."write-only") -> (refnum out=w391:refnum<file>)  [unwired: 3 in, 2 out]
            n225 = Open/Create/Replace File(file path (use dialog)=w429, operation (0:open)=T4."create", access (0:read/write)=enum16{"read/write", "read-only", "write-only"}."write-only") -> (refnum out=w414:refnum<file>)  [unwired: 3 in, 2 out]
            n226 = Open/Create/Replace File(file path (use dialog)=w395, operation (0:open)=T4."create", access (0:read/write)=enum16{"read/write", "read-only", "write-only"}."write-only") -> (refnum out=w390:refnum<file>)  [unwired: 3 in, 2 out]
            n227 = Write to Binary File(file (use dialog)=w365, data=w367) -> (refnum out=w364:refnum<file>)  [unwired: 4 in, 2 out]
            n228 = Write to Binary File(file (use dialog)=w388, data=w387) -> (refnum out=w386:refnum<file>)  [unwired: 4 in, 2 out]
            n229 = local write "Heading (deg)"(w389) -> ()
            n230 = local write "H"(w389) -> ()
          }
          frame #3 {
            n231 = call-poly <vilib>:"DAQmx Create Virtual Channel.vi"("lines"=tag "Dev1/port0/line3") -> ("task out"=w568:refnum<k21>)  [unwired: 13 in, 1 out]
            n232 = call-poly <vilib>:"DAQmx Create Virtual Channel.vi"("lines"=tag "Dev1/port0/line2") -> ("task out"=w569:refnum<k21>)  [unwired: 13 in, 1 out]
            n233 = call-poly <vilib>:"DAQmx Create Virtual Channel.vi"("lines"=tag "Dev1/port0/line6") -> ("task out"=w561:refnum<k21>)  [unwired: 13 in, 1 out]
            n234 = call-poly <vilib>:"DAQmx Create Virtual Channel.vi"("physical channels"=tag "Dev1/ao0") -> ("task out"=w557:refnum<k21>)  [unwired: 13 in, 1 out]
            n235 = Reciprocal(x="Data Rate (Hz)") -> (1/x=w586:dbl)
            n236 = call-poly <vilib>:"DAQmx Create Virtual Channel.vi"("lines"=tag "Dev1/port0/line1") -> ("task out"=w564:refnum<k21>)  [unwired: 13 in, 1 out]
            n237 = node-c288(w586) -> (w588:T8)  [unwired: 3 in]
            n238 = timed-loop {
              timing: w588 -> [_]
              timing-out: [_] -> w587
              tunnel: w584 -> [w671]
              tunnel: w583 -> [w672]
              tunnel: w582 -> [w670]
              shift-right: [w653] -> w578
              shift-left: w569 -> [w655]
              shift-right: [w654] -> w579
              shift-left: w568 -> [w656]
              tunnel: w581 -> [w669]
              tunnel: [w668] -> w580
              shift-right: [w665] -> _
              shift-left: w563 -> [w666]
              tunnel: w577 -> [w664]
              tunnel: [w663] -> w576
              tunnel: [w662] -> w575
              tunnel: w574 -> [w661]
              tunnel: w573 -> [w660]
              tunnel: w572 -> [w659]
              tunnel: [w658] -> w571
              tunnel: [w657] -> w570
              shift-right: [w649] -> _
              shift-left: w564 -> [w652]
              shift-right: [w600] -> _
              shift-left: _ -> [w607]
              shift-right: [w602] -> w560
              shift-left: w561 -> [w605]
              shift-right: [w591] -> w556
              shift-left: w557 -> [w592]
              i -> [w667]
              stop <- w646 stop-if-true
              w635 = T14 {"Search Direction"=0, "Edge Options"={"Edge Polarity"=0, "Kernel Size"=3, "Width"=3, "Minimum Edge Strength"=2.0, "Interpolation Type"=enum."Bilinear Fixed", "Data Processing Method"=enum."Average"}, "Show Search Area"=TRUE, "Show Search Lines"=TRUE, "Show Edges Found"=TRUE, "Show Result"=TRUE, "Search Area Color"=65280, "Search Lines Color"=255, "Edge Locations Color"=16776960, "Result Color"=16711680, "Overlay Group Name"=""} ("Options")
              n239 = node-c288() -> ()  [unwired: 1 in, 1 out]
              n240 = To Double Precision Float(number=w667) -> (double precision float=w611:dbl)
              n241 = local read "Wind Trial?"() -> (w590:bool)
              n242 = local read "Data Rate (Hz)"() -> (w626:dbl)
              n243 = local read "Trial Light"() -> (w589:dbl)
              n244 = Increment(x=w611) -> (x+1=w622:dbl)
              n245 = call <vilib>:"DAQmx Start Task.vi"("task/channels in"=w592) -> ("task out"=w594:refnum<k21>)  [unwired: 13 in, 1 out]
              n246 = call <vilib>:"DAQmx Start Task.vi"("task/channels in"=w605) -> ("task out"=w604:refnum<k21>)  [unwired: 13 in, 1 out]
              n247 = call <vilib>:"DAQmx Start Task.vi"("task/channels in"=w652) -> ("task out"=w651:refnum<k21>)  [unwired: 13 in, 1 out]
              n248 = Divide(x=w622, y=w626) -> (x/y=w625:dbl)
              n249 = call-poly <vilib>:"DAQmx Write.vi"("task/channels in"=w594, "data"=w589) -> ("task out"=w593:refnum<k21>)  [unwired: 11 in, 2 out]
              n250 = call-poly <vilib>:"DAQmx Write.vi"("task/channels in"=w604, "data"=w590) -> ("task out"=w603:refnum<k21>)  [unwired: 11 in, 2 out]
              n251 = call "IMAQ Create"("Image Name"="flyim") -> ("New Image"=w645:T3)  [unwired: 3 in, 2 out]
              n252 = Greater?(x=w625, y="Trial Duration (s)") -> (0:→"Trial End":bool)
              n253 = call <vilib>:"DAQmx Stop Task.vi"("task/channels in"=w593) -> ("task out"=w591:refnum<k21>)  [unwired: 13 in, 1 out]
              n254 = call <vilib>:"DAQmx Stop Task.vi"("task/channels in"=w603) -> ("task out"=w602:refnum<k21>)  [unwired: 13 in, 1 out]
              n255 = call-poly <vilib>:"DAQmx Read.vi"("task/channels in"=w651) -> ("task out"=w650:refnum<k21>, "data"=→"Motor Error":bool)  [unwired: 12 in, 1 out]
              n256 = call <vilib>:"IMAQdx Grab.vi"("Wait for Next Buffer? (Yes)"=FALSE, "Image In"=w645, "Session In"=w672) -> ("Image Out"=w636:T3)  [unwired: 1 in, 7 out]
              n257 = call "IMAQ Threshold"("Keep/Replace Value (Replace)"=FALSE, "Range"="Image Threshold", "Image Src"=w636) -> ("Image Dst Out"=w641:T3)  [unwired: 7 in, 1 out]
              n258 = call <vilib>:"DAQmx Stop Task.vi"("task/channels in"=w650) -> ("task out"=w649:refnum<k21>)  [unwired: 13 in, 1 out]
              n259 = call "IMAQ Find Edge"("Line Fit Options"="L options", "Options"=w635, "ROI Descriptor"=w671, "Image"=w641) -> ("Straight Edges"=w638:T15, "Image Out"=w640:T3)  [unwired: 4 in, 2 out]
              n260 = call "IMAQ Find Edge"("Line Fit Options"="R options", "Options"=w635, "ROI Descriptor"=w670, "Image"=w640) -> ("Straight Edges"=w637:T15, "Image Out"=→"Image":T3)  [unwired: 4 in, 2 out]
              n261 = Array To Cluster(array=w637) -> (cluster=w628:T16)
              n262 = Array To Cluster(array=w638) -> (cluster=w627:T16)
              n263 = Unbundle By Name(w628) -> ("Straight Edges[0].Angle (Pixel)"=w633:dbl)
              n264 = Unbundle By Name(w627) -> ("Straight Edges[0].Angle (Pixel)"=w634:dbl)
              n265 = Absolute Value(x=w633) -> (abs(x)=w612:dbl)
              "L WBA" <- w612
              n266 = Absolute Value(x=w634) -> (abs(x)=w613:dbl)
              "R WBA" <- w613
              n267 = Write to Binary File(file (use dialog)=w659, data=w613) -> (refnum out=w658:refnum<file>)  [unwired: 4 in, 2 out]
              n268 = Write to Binary File(file (use dialog)=w660, data=w612) -> (refnum out=w657:refnum<file>)  [unwired: 4 in, 2 out]
              n269 = Subtract(x=w612, y=w613) -> (x-y=w631:dbl)
              "L-R WBA" <- w631
              n270 = case shown="False" "Reversed Tether?" {
                tunnel: w631 -> [w675 w677]
                tunnel: [w674 w676] -> w630
                tunnel: "L-R WBA Offset (deg)" -> [w673 w678]
                frame False {
                  n271 = Add ("Add.vi")(x=w675, y=w673) -> (x+y=w674:dbl)
                }
                frame True {
                  n272 = Subtract(x=w677, y=w678) -> (x-y=w676:dbl)
                }
              }
              n273 = Multiply(x=w630, y="deltaWBA Scale Factor (k, unitless)") -> (x*y=w632:dbl)
              n274 = case shown="False" "Reversed Tether?" {
                tunnel: w632 -> [w680 w681]
                tunnel: [w679 w681] -> w598
                frame False {
                  n275 = Negate(x=w680) -> (-x=w679:dbl)
                }
                frame True {
                }
              }
              "Scaled deltaWBA (deg)" <- w598
              "deltaWBA" <- w598
              n276 = Greater Or Equal To 0?(x=w598) -> (x >= 0?=w599:bool)
              n277 = case shown="False" w599 {
                tunnel: [w692 w709] -> w600
                tunnel: "Max steps/sample" -> [w691 w705]
                tunnel: w598 -> [w685 w704]
                frame False {
                  n278 = Absolute Value(x=w685) -> (abs(x)=w686:dbl)
                  n279 = Quotient & Remainder(x=w686, y=0.36) -> (x-y*floor(x/y)=w684:dbl, floor(x/y)=w687:dbl)
                  n280 = Greater?(x=w684, y=0.18) -> (0:w688:bool)
                  n281 = Negate(x=w691) -> (-x=w693:dbl)
                  n282 = case shown="True" w688 {
                    tunnel: w687 -> [w695 w698]
                    tunnel: [w695 w696] -> w683
                    frame False {
                    }
                    frame True {
                      n283 = Add(x=w698, y=1.0) -> (x+y=w696:dbl)
                    }
                  }
                  n284 = Negate(x=w683) -> (-x=w682:dbl)
                  n285 = Less?(x=w682, y=w693) -> (x < y?=w694:bool)
                  n286 = case shown="False" w694 {
                    tunnel: w693 -> [_ w700]
                    tunnel: [w699 w700] -> w692
                    tunnel: w682 -> [w699 _]
                    frame False {
                    }
                    frame True {
                    }
                  }
                }
                frame True {
                  n287 = Quotient & Remainder(x=w704, y=0.36) -> (x-y*floor(x/y)=w702:dbl, floor(x/y)=w707:dbl)
                  n288 = Greater?(x=w702, y=0.18) -> (0:w703:bool)
                  n289 = case shown="True" w703 {
                    tunnel: w707 -> [w711 w714]
                    tunnel: [w711 w712] -> w708
                    frame False {
                    }
                    frame True {
                      n290 = Add(x=w714, y=1.0) -> (x+y=w712:dbl)
                    }
                  }
                  n291 = Greater?(x=w708, y=w705) -> (0:w710:bool)
                  n292 = case shown="False" w710 {
                    tunnel: w705 -> [_ w716]
                    tunnel: [w715 w716] -> w709
                    tunnel: w708 -> [w715 _]
                    frame False {
                    }
                    frame True {
                    }
                  }
                }
              }
              "X (steps/sample)" <- w600
              "X (steps/sample)" <- w600
              n293 = Multiply(x=0.36 ("y"), y=w600) -> (x*y=w614:dbl)
              n294 = Add ("Add.vi")(x=w614, y=w666) -> (x+y=w618:dbl)
              n295 = Add(x=w618, y=180.0 ("x")) -> (x+y=w619:dbl)
              n296 = Quotient & Remainder(x=w619, y=360.0) -> (x-y*floor(x/y)=w620:dbl)  [unwired: 1 out]
              n297 = Subtract(x=w620, y=180.0) -> (x-y=w665:dbl)
              "H" <- w665
              "Heading (deg)" <- w665
              n298 = Write to Binary File(file (use dialog)=w664, data=w665) -> (refnum out=w663:refnum<file>)  [unwired: 4 in, 2 out]
              n299 = Write to Binary File(file (use dialog)=w661, data=w598) -> (refnum out=w668:refnum<file>)  [unwired: 4 in, 2 out]
              n300 = Write to Binary File(file (use dialog)=w669, data=w600) -> (refnum out=w662:refnum<file>)  [unwired: 4 in, 2 out]
              n301 = Not Equal To 0?(x=w607) -> (x != 0?=w608:bool)
              n302 = case shown="True" w608 {
                tunnel: w656 -> [w718 w725]
                tunnel: w655 -> [w717 w724]
                tunnel: w607 -> [_ w723]
                tunnel: [w717 w722] -> w653
                tunnel: [w718 w721] -> w654
                frame False {
                }
                frame True {
                  n303 = Reciprocal(x="Step Rate (Hz)") -> (1/x=w719:dbl)
                  n304 = node-c288(w719) -> (w727:T8)  [unwired: 3 in]
                  n305 = timed-loop {
                    timing: w727 -> [_]
                    timing-out: [_] -> w726
                    tunnel: w723 -> [w741]
                    shift-right: [w734] -> w721
                    shift-left: w725 -> [w738]
                    shift-right: [w733] -> w722
                    shift-left: w724 -> [w736]
                    i -> [w732]
                    stop <- w730 stop-if-true
                    n306 = node-c288() -> ()  [unwired: 1 in, 1 out]
                    n307 = To Double Precision Float(number=w732) -> (double precision float=w731:dbl)
                    n308 = Absolute Value(x=w741) -> (abs(x)=w740:dbl)
                    n309 = call <vilib>:"DAQmx Start Task.vi"("task/channels in"=w738) -> ("task out"=w737:refnum<k21>)  [unwired: 13 in, 1 out]
                    n310 = call <vilib>:"DAQmx Start Task.vi"("task/channels in"=w736) -> ("task out"=w735:refnum<k21>)  [unwired: 13 in, 1 out]
                    n311 = Increment(x=w731) -> (x+1=w739:dbl)
                    n312 = Greater Than 0?(x=w741) -> (x > 0?=w742:bool)
                    n313 = Equal?(x=w740, y=w739) -> (x = y?=w729:bool)
                    n314 = case shown="False" w742 {
                      tunnel: [w745 w765] -> w734
                      tunnel: [w746 w766] -> w733
                      tunnel: w735 -> [w748 w768]
                      tunnel: w737 -> [w747 w767]
                      frame True {
                        n315 = flat-sequence {
                          tunnel: w748 -> [w756]
                          tunnel: w747 -> [w755]
                          tunnel: [w751] -> w744
                          tunnel: [w749] -> w743
                          tunnel: [w762] -> w745
                          tunnel: [w758] -> w746
                          tunnel: w744 -> [w761]
                          tunnel: w743 -> [w762]
                          frame #0 {
                            n316 = call-poly <vilib>:"DAQmx Write.vi"("task/channels in"=w755, "data"=FALSE) -> ("task out"=w750:refnum<k21>)  [unwired: 11 in, 2 out]
                            n317 = call-poly <vilib>:"DAQmx Write.vi"("task/channels in"=w756, "data"=TRUE) -> ("task out"=w752:refnum<k21>)  [unwired: 11 in, 2 out]
                            n318 = call <vilib>:"DAQmx Stop Task.vi"("task/channels in"=w750) -> ("task out"=w749:refnum<k21>)  [unwired: 13 in, 1 out]
                            n319 = call <vilib>:"DAQmx Stop Task.vi"("task/channels in"=w752) -> ("task out"=w751:refnum<k21>)  [unwired: 13 in, 1 out]
                          }
                          frame #1 {
                            n320 = call <vilib>:"DAQmx Start Task.vi"("task/channels in"=w761) -> ("task out"=w760:refnum<k21>)  [unwired: 13 in, 1 out]
                            n321 = call-poly <vilib>:"DAQmx Write.vi"("task/channels in"=w760, "data"=FALSE) -> ("task out"=w759:refnum<k21>)  [unwired: 11 in, 2 out]
                            n322 = call <vilib>:"DAQmx Stop Task.vi"("task/channels in"=w759) -> ("task out"=w758:refnum<k21>)  [unwired: 13 in, 1 out]
                          }
                        }
                      }
                      frame False {
                        n323 = flat-sequence {
                          tunnel: w768 -> [w776]
                          tunnel: w767 -> [w775]
                          tunnel: [w771] -> w764
                          tunnel: [w769] -> w763
                          tunnel: [w778] -> w765
                          tunnel: [w777] -> w766
                          tunnel: w764 -> [w777]
                          tunnel: w763 -> [w779]
                          frame #0 {
                            n324 = call-poly <vilib>:"DAQmx Write.vi"("task/channels in"=w775, "data"=TRUE) -> ("task out"=w770:refnum<k21>)  [unwired: 11 in, 2 out]
                            n325 = call-poly <vilib>:"DAQmx Write.vi"("task/channels in"=w776, "data"=FALSE) -> ("task out"=w772:refnum<k21>)  [unwired: 11 in, 2 out]
                            n326 = call <vilib>:"DAQmx Stop Task.vi"("task/channels in"=w770) -> ("task out"=w769:refnum<k21>)  [unwired: 13 in, 1 out]
                            n327 = call <vilib>:"DAQmx Stop Task.vi"("task/channels in"=w772) -> ("task out"=w771:refnum<k21>)  [unwired: 13 in, 1 out]
                          }
                          frame #1 {
                            n328 = call <vilib>:"DAQmx Start Task.vi"("task/channels in"=w779) -> ("task out"=w782:refnum<k21>)  [unwired: 13 in, 1 out]
                            n329 = call-poly <vilib>:"DAQmx Write.vi"("task/channels in"=w782, "data"=FALSE) -> ("task out"=w781:refnum<k21>)  [unwired: 11 in, 2 out]
                            n330 = call <vilib>:"DAQmx Stop Task.vi"("task/channels in"=w781) -> ("task out"=w778:refnum<k21>)  [unwired: 13 in, 1 out]
                          }
                        }
                      }
                    }
                    n331 = local read "Motor Error"() -> (w728:bool)
                    n332 = Or(x=w729, y=w728) -> (x .or. y?=w730:bool)
                    n333 = node-c288() -> ()  [unwired: 1 in, 1 out]
                  }
                  n334 = node-c288(w726) -> ()  [unwired: 1 out]
                }
              }
              n335 = local read "Motor Error"() -> (w647:bool)
              n336 = local read "Trial End"() -> (w648:bool)
              n337 = Or(x=w648, y=w647) -> (x .or. y?=w646:bool)
              n338 = node-c288() -> ()  [unwired: 1 in, 1 out]
            }
            n339 = node-c288(w587) -> ()  [unwired: 1 out]
          }
          frame #4 {
            n340 = local read "H"() -> (w807:dbl)
            n341 = Absolute Value(x=w807) -> (abs(x)=w801:dbl)
            n342 = Close File(refnum=w818) -> ()  [unwired: 1 in, 2 out]
            n343 = Close File(refnum=w817) -> ()  [unwired: 1 in, 2 out]
            n344 = Close File(refnum=w816) -> ()  [unwired: 1 in, 2 out]
            n345 = Close File(refnum=w815) -> ()  [unwired: 1 in, 2 out]
            n346 = Close File(refnum=w819) -> ()  [unwired: 1 in, 2 out]
            n347 = Greater Than 0?(x=w807) -> (x > 0?=w814:bool)
            n348 = To Long Integer(number=w801) -> (32bit integer=w800:i32)
            n349 = Not Equal To 0?(x=w800) -> (x != 0?=w813:bool)
            n350 = case shown="True" w813 {
              tunnel: w821 -> [_ w825]
              tunnel: w820 -> [_ w824]
              tunnel: w814 -> [_ w823]
              tunnel: w807 -> [_ w822]
              frame False {
              }
              frame True {
                n351 = case shown="False" w823 {
                  tunnel: w825 -> [w836 w887]
                  tunnel: w824 -> [w835 w886]
                  tunnel: w822 -> [w833 w884]
                  frame True {
                    n352 = local read "X (steps/sample)"() -> (w827:dbl)
                    n353 = Divide(x=w833, y=0.36) -> (x/y=w829:dbl)
                    n354 = Add(x=1.0, y=w827) -> (x+y=w828:dbl)
                    n355 = Subtract(x=w829, y=w828) -> (x-y=w831:dbl)
                    n356 = local read "Step Rate (Hz)"() -> (w834:dbl)
                    n357 = Reciprocal(x=w834) -> (1/x=w837:dbl)
                    n358 = node-c288(w837) -> (w839:T8)  [unwired: 3 in]
                    n359 = Absolute Value(x=w831) -> (abs(x)=w830:dbl)
                    n360 = timed-loop {
                      timing: w839 -> [_]
                      timing-out: [_] -> w838
                      shift-right: [w851] -> _
                      shift-left: w835 -> [w849]
                      shift-right: [w852] -> _
                      shift-left: w836 -> [w850]
                      tunnel: w830 -> [w843]
                      i -> [w841]
                      stop <- w846 stop-if-true
                      n361 = node-c288() -> ()  [unwired: 1 in, 1 out]
                      n362 = To Long Integer(number=w841) -> (32bit integer=w840:i32)
                      n363 = To Long Integer(number=w843) -> (32bit integer=w842:i32)
                      n364 = flat-sequence {
                        tunnel: w850 -> [w859]
                        tunnel: w849 -> [w857]
                        tunnel: [w862] -> w848
                        tunnel: [w860] -> w847
                        tunnel: [w869] -> w851
                        tunnel: [w864] -> w852
                        tunnel: w848 -> [w867]
                        tunnel: w847 -> [w869]
                        frame #0 {
                          n365 = call <vilib>:"DAQmx Start Task.vi"("task/channels in"=w859) -> ("task out"=w858:refnum<k21>)  [unwired: 13 in, 1 out]
                          n366 = call <vilib>:"DAQmx Start Task.vi"("task/channels in"=w857) -> ("task out"=w856:refnum<k21>)  [unwired: 13 in, 1 out]
                          n367 = call-poly <vilib>:"DAQmx Write.vi"("task/channels in"=w858, "data"=TRUE) -> ("task out"=w863:refnum<k21>)  [unwired: 11 in, 2 out]
                          n368 = call-poly <vilib>:"DAQmx Write.vi"("task/channels in"=w856, "data"=FALSE) -> ("task out"=w861:refnum<k21>)  [unwired: 11 in, 2 out]
                          n369 = call <vilib>:"DAQmx Stop Task.vi"("task/channels in"=w863) -> ("task out"=w862:refnum<k21>)  [unwired: 13 in, 1 out]
                          n370 = call <vilib>:"DAQmx Stop Task.vi"("task/channels in"=w861) -> ("task out"=w860:refnum<k21>)  [unwired: 13 in, 1 out]
                        }
                        frame #1 {
                          n371 = call <vilib>:"DAQmx Start Task.vi"("task/channels in"=w867) -> ("task out"=w866:refnum<k21>)  [unwired: 13 in, 1 out]
                          n372 = call-poly <vilib>:"DAQmx Write.vi"("task/channels in"=w866, "data"=FALSE) -> ("task out"=w865:refnum<k21>)  [unwired: 11 in, 2 out]
                          n373 = call <vilib>:"DAQmx Stop Task.vi"("task/channels in"=w865) -> ("task out"=w864:refnum<k21>)  [unwired: 13 in, 1 out]
                        }
                      }
                      n374 = Increment(x=w840) -> (x+1=w853:i32)
                      n375 = Equal?(x=w842, y=w853) -> (x = y?=w844:bool)
                      n376 = local read "Motor Error"() -> (w845:bool)
                      n377 = Or(x=w845, y=w844) -> (x .or. y?=w846:bool)
                      n378 = node-c288() -> ()  [unwired: 1 in, 1 out]
                    }
                    n379 = node-c288(w838) -> ()  [unwired: 1 out]
                  }
                  frame False {
                    n380 = local read "X (steps/sample)"() -> (w879:dbl)
                    n381 = Divide(x=w884, y=0.36) -> (x/y=w882:dbl)
                    n382 = Add(x=1.0, y=w879) -> (x+y=w877:dbl)
                    n383 = local read "Step Rate (Hz)"() -> (w885:dbl)
                    n384 = Reciprocal(x=w885) -> (1/x=w888:dbl)
                    n385 = node-c288(w888) -> (w890:T8)  [unwired: 3 in]
                    n386 = Subtract(x=w882, y=w877) -> (x-y=w881:dbl)
                    n387 = Absolute Value(x=w881) -> (abs(x)=w880:dbl)
                    n388 = timed-loop {
                      timing: w890 -> [_]
                      timing-out: [_] -> w889
                      shift-right: [w902] -> _
                      shift-left: w886 -> [w900]
                      shift-right: [w903] -> _
                      shift-left: w887 -> [w901]
                      tunnel: w880 -> [w892]
                      i -> [w894]
                      stop <- w897 stop-if-true
                      n389 = node-c288() -> ()  [unwired: 1 in, 1 out]
                      n390 = To Long Integer(number=w892) -> (32bit integer=w891:i32)
                      n391 = To Long Integer(number=w894) -> (32bit integer=w893:i32)
                      n392 = flat-sequence {
                        tunnel: w901 -> [w910]
                        tunnel: w900 -> [w908]
                        tunnel: [w913] -> w899
                        tunnel: [w911] -> w898
                        tunnel: [w916] -> w902
                        tunnel: [w915] -> w903
                        tunnel: w899 -> [w915]
                        tunnel: w898 -> [w917]
                        frame #0 {
                          n393 = call <vilib>:"DAQmx Start Task.vi"("task/channels in"=w910) -> ("task out"=w909:refnum<k21>)  [unwired: 13 in, 1 out]
                          n394 = call <vilib>:"DAQmx Start Task.vi"("task/channels in"=w908) -> ("task out"=w907:refnum<k21>)  [unwired: 13 in, 1 out]
                          n395 = call-poly <vilib>:"DAQmx Write.vi"("task/channels in"=w909, "data"=FALSE) -> ("task out"=w914:refnum<k21>)  [unwired: 11 in, 2 out]
                          n396 = call-poly <vilib>:"DAQmx Write.vi"("task/channels in"=w907, "data"=TRUE) -> ("task out"=w912:refnum<k21>)  [unwired: 11 in, 2 out]
                          n397 = call <vilib>:"DAQmx Stop Task.vi"("task/channels in"=w914) -> ("task out"=w913:refnum<k21>)  [unwired: 13 in, 1 out]
                          n398 = call <vilib>:"DAQmx Stop Task.vi"("task/channels in"=w912) -> ("task out"=w911:refnum<k21>)  [unwired: 13 in, 1 out]
                        }
                        frame #1 {
                          n399 = call <vilib>:"DAQmx Start Task.vi"("task/channels in"=w917) -> ("task out"=w919:refnum<k21>)  [unwired: 13 in, 1 out]
                          n400 = call-poly <vilib>:"DAQmx Write.vi"("task/channels in"=w919, "data"=FALSE) -> ("task out"=w918:refnum<k21>)  [unwired: 11 in, 2 out]
                          n401 = call <vilib>:"DAQmx Stop Task.vi"("task/channels in"=w918) -> ("task out"=w916:refnum<k21>)  [unwired: 13 in, 1 out]
                        }
                      }
                      n402 = Increment(x=w893) -> (x+1=w904:i32)
                      n403 = Equal?(x=w891, y=w904) -> (x = y?=w896:bool)
                      n404 = local read "Motor Error"() -> (w895:bool)
                      n405 = Or(x=w895, y=w896) -> (x .or. y?=w897:bool)
                      n406 = node-c288() -> ()  [unwired: 1 in, 1 out]
                    }
                    n407 = node-c288(w889) -> ()  [unwired: 1 out]
                  }
                }
              }
            }
            n408 = call <vilib>:"DAQmx Start Task.vi"("task/channels in"=w804) -> ("task out"=w806:refnum<k21>)  [unwired: 13 in, 1 out]
            n409 = call <vilib>:"DAQmx Start Task.vi"("task/channels in"=w811) -> ("task out"=w810:refnum<k21>)  [unwired: 13 in, 1 out]
            n410 = call-poly <vilib>:"DAQmx Write.vi"("task/channels in"=w806, "data"=0.0) -> ("task out"=w805:refnum<k21>)  [unwired: 11 in, 2 out]
            n411 = call-poly <vilib>:"DAQmx Write.vi"("task/channels in"=w810, "data"=FALSE) -> ("task out"=w809:refnum<k21>)  [unwired: 11 in, 2 out]
            n412 = call <vilib>:"DAQmx Stop Task.vi"("task/channels in"=w805) -> ()  [unwired: 13 in, 2 out]
            n413 = call <vilib>:"DAQmx Stop Task.vi"("task/channels in"=w809) -> ()  [unwired: 13 in, 2 out]
          }
          frame #5 {
            n414 = Unbundle(w945) -> ("y"=w939:i32, "y"=w938:i32, "y"=w937:i32, "y"=w936:i32, "y"=w932:i32, "y"=w931:i32)
            n415 = Greater?(x=w935, y=3.0) -> (0:w933:bool)
            n416 = case shown="True" w933 {
              tunnel: [w966 w1017] -> w944
              tunnel: [w965 w1016] -> w943
              tunnel: [w964 w1015] -> w942
              tunnel: [w963 w1014] -> w941
              tunnel: w939 -> [w962 w1013]
              tunnel: w938 -> [w961 w1012]
              tunnel: w937 -> [w960 w1011]
              tunnel: w936 -> [w959 w1010]
              tunnel: w935 -> [w952 w1003]
              tunnel: w932 -> [w956 w1007]
              tunnel: w931 -> [w955 w1006]
              tunnel: [w954 w1005] -> w930
              tunnel: [w953 w1004] -> w929
              frame True {
                n417 = Greater?(x=w952, y=4.0) -> (0:w957:bool)
                n418 = case shown="True" w957 {
                  tunnel: w962 -> [w967 w986]
                  tunnel: w961 -> [w968 w985]
                  tunnel: w960 -> [w969 w984]
                  tunnel: w959 -> [w972 w983]
                  tunnel: [w967 w979] -> w966
                  tunnel: [w968 w980] -> w965
                  tunnel: [w969 w982] -> w964
                  tunnel: [w973 w981] -> w963
                  tunnel: w952 -> [_ w978]
                  tunnel: w956 -> [w970 w977]
                  tunnel: w955 -> [w971 w976]
                  tunnel: [w970 w975] -> w954
                  tunnel: [w971 w974] -> w953
                  frame False {
                    n419 = Increment(x=w972) -> (x+1=w973:i32)
                  }
                  frame True {
                    n420 = Greater?(x=w978, y=5.0) -> (0:w987:bool)
                    n421 = case shown="True" w987 {
                      tunnel: w986 -> [w995 w1002]
                      tunnel: w985 -> [w994 w1001]
                      tunnel: w984 -> [w992 w1000]
                      tunnel: w983 -> [w993 w998]
                      tunnel: [w995 w1002] -> w979
                      tunnel: [w994 w1001] -> w980
                      tunnel: [w992 w1000] -> w982
                      tunnel: [w993 w998] -> w981
                      tunnel: w977 -> [w991 w999]
                      tunnel: w976 -> [w989 w997]
                      tunnel: [w990 w999] -> w975
                      tunnel: [w989 w996] -> w974
                      frame False {
                        n422 = Increment(x=w991) -> (x+1=w990:i32)
                      }
                      frame True {
                        n423 = Increment(x=w997) -> (x+1=w996:i32)
                      }
                    }
                  }
                }
              }
              frame False {
                n424 = Greater?(x=w1003, y=1.0) -> (0:w1008:bool)
                n425 = case shown="True" w1008 {
                  tunnel: w1013 -> [w1019 w1037]
                  tunnel: w1012 -> [w1021 w1036]
                  tunnel: w1011 -> [w1022 w1035]
                  tunnel: w1010 -> [w1020 w1034]
                  tunnel: [w1018 w1030] -> w1017
                  tunnel: [w1021 w1031] -> w1016
                  tunnel: [w1022 w1033] -> w1015
                  tunnel: [w1020 w1032] -> w1014
                  tunnel: w1003 -> [_ w1029]
                  tunnel: w1007 -> [w1023 w1028]
                  tunnel: w1006 -> [w1024 w1027]
                  tunnel: [w1023 w1026] -> w1005
                  tunnel: [w1024 w1025] -> w1004
                  frame False {
                    n426 = Increment(x=w1019) -> (x+1=w1018:i32)
                  }
                  frame True {
                    n427 = Greater?(x=w1029, y=2.0) -> (0:w1038:bool)
                    n428 = case shown="False" w1038 {
                      tunnel: w1037 -> [w1046 w1053]
                      tunnel: w1036 -> [w1041 w1052]
                      tunnel: w1035 -> [w1044 w1047]
                      tunnel: w1034 -> [w1045 w1050]
                      tunnel: [w1046 w1053] -> w1030
                      tunnel: [w1040 w1052] -> w1031
                      tunnel: [w1044 w1048] -> w1033
                      tunnel: [w1045 w1050] -> w1032
                      tunnel: w1028 -> [w1042 w1051]
                      tunnel: w1027 -> [w1043 w1049]
                      tunnel: [w1042 w1051] -> w1026
                      tunnel: [w1043 w1049] -> w1025
                      frame False {
                        n429 = Increment(x=w1041) -> (x+1=w1040:i32)
                      }
                      frame True {
                        n430 = Increment(x=w1047) -> (x+1=w1048:i32)
                      }
                    }
                  }
                }
              }
            }
            n431 = call-poly <vilib>:"DAQmx Create Virtual Channel.vi"("lines"=tag "Dev1/port0/line0") -> ("task out"=w950:refnum<k21>)  [unwired: 13 in, 1 out]
            n432 = call <vilib>:"DAQmx Start Task.vi"("task/channels in"=w950) -> ("task out"=w949:refnum<k21>)  [unwired: 13 in, 1 out]
            n433 = call-poly <vilib>:"DAQmx Write.vi"("task/channels in"=w949, "data"=TRUE) -> ("task out"=w948:refnum<k21>)  [unwired: 11 in, 2 out]
            n434 = call <vilib>:"DAQmx Stop Task.vi"("task/channels in"=w948) -> ()  [unwired: 13 in, 2 out]
          }
        }
        n435 = Increment(x=w244) -> (x+1=w234:i32)
        "Trial" <- w234
        n436 = Divide(x=w234, y=w235) -> (x/y=→"Slide":dbl)
        "V, 0" <- w215
        "M, 0" <- w213
        "W, 0" <- w211
        "V, 90" <- w209
        "M, 90" <- w173
        "W, 90" <- w174
      }
    }
    frame #3 {
      n437 = Close File(refnum=w1055) -> ()  [unwired: 1 in, 2 out]
      n438 = Close File(refnum=w1061) -> ()  [unwired: 1 in, 2 out]
      n439 = call-poly <vilib>:"DAQmx Create Virtual Channel.vi"("physical channels"=tag "Dev1/ao1") -> ("task out"=w1058:refnum<k21>)  [unwired: 13 in, 1 out]
      n440 = Close File(refnum=w1054) -> ()  [unwired: 1 in, 2 out]
      n441 = call <vilib>:"DAQmx Start Task.vi"("task/channels in"=w1058) -> ("task out"=w1060:refnum<k21>)  [unwired: 13 in, 1 out]
      n442 = call-poly <vilib>:"DAQmx Write.vi"("task/channels in"=w1060, "data"=5.0) -> ("task out"=w1059:refnum<k21>)  [unwired: 11 in, 2 out]
      n443 = call <vilib>:"DAQmx Stop Task.vi"("task/channels in"=w1059) -> ()  [unwired: 13 in, 2 out]
    }
  }
